vi "Write Flow Control Valve Setpoint.vi"(10 "Flow Control Valve Setpoint":dbl[unit], 11 "IActuatorCylinder in":refnum<class "ILCControlledActuatorCylinder.lvclass">) -> (3 "IActuatorCylinder out":refnum<class "ILCControlledActuatorCylinder.lvclass">)   [LabVIEW 2015, in "ILCControlledActuatorCylinder.lvclass"]
uses:
  ILCControlledActuatorCylinder.lvclass
  ILCControlledActuatorCylinder.lvclass/ILCControlledActuatorCylinder.ctl
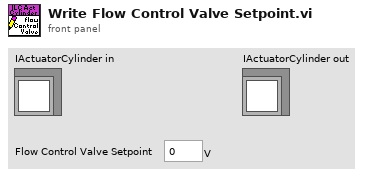
[diagram p1: front panel]
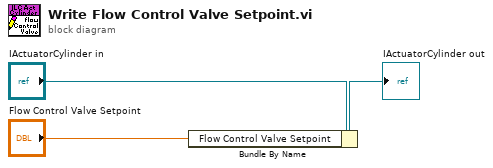
[diagram p0: block diagram]
diagram:
  n1 = Bundle By Name(cluster="IActuatorCylinder in", "Flow Control Valve Setpoint"="Flow Control Valve Setpoint") -> (→"IActuatorCylinder out":refnum<class "ILCControlledActuatorCylinder.lvclass">)
